vi "DMM Read (Simulate).vi"(8 "error in (no error)":errorcluster, 11 "Instrument Refnum in":refnum<visa-resource-name>) -> (0 "error out":errorcluster, 2 "Measurement":dbl, 3 "Instrument Refnum out":refnum<visa-resource-name>)   [LabVIEW 2012]
doc: "Simulates reading a simgle measurement from a DMM"
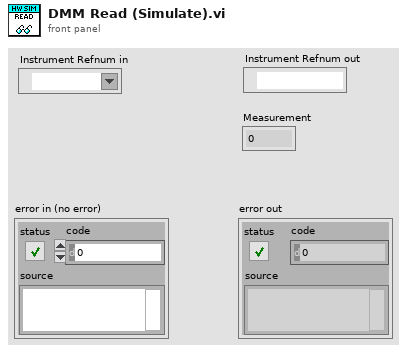
[diagram p1: front panel]
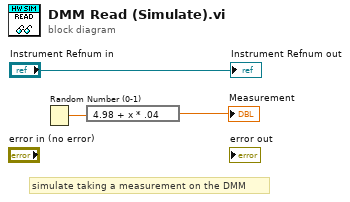
[diagram p0: block diagram]
diagram:
  # "simulate taking a measurement on the DMM"
  n1 = Random Number (0-1)() -> (number: 0 to 1=w2:dbl)
  n2 = expression code="4.98 + x * .04"(w2) -> (→"Measurement":dbl)
  "Instrument Refnum out" <- "Instrument Refnum in"
